vi "ShuffleSplit.vi"(6 "Groups":string[][](array[string]), 8 "error in (no error)":errorcluster caption="entrée d'erreur (pas d'erreur)", 9 "y":string[][](array[string]), 10 "X":string[][](array[string]), 11 "ShuffleSplit":T2={"n_splits"=10, "test_size"="None", "train_size"="None", "random_state"=-1} {"random_state" min=-1}) -> (0 "error out":errorcluster caption="sortie d'erreur", 3 "Split":T1(array[cluster]))   [LabVIEW 2020]
doc: "Random permutation cross-validator\n\nYields indices to split data into training and test sets.\n\nNote: contrary to other cross-validation strategies, random splits do not guarantee that all folds will be different, although this is still very likely for sizeable datasets.\n\n\nParameters :\n\n- n_splits : int, default=10\nNumber of re-shuffling & splitting iterations.\n\n- test_size : float or int, default=None\nIf float, should be between 0.0 and 1.0 and represent the proportion of the dataset to include in the test split. If int, represents the absolute number of test samples. If None, the value is set to the complement of the train size. If train_size is also None, it will be set to 0.1.\n\n- train_size : float or int, default=None\nIf float, should be between 0.0 and 1.0 and represent the proportion of the dataset to include in the train split. If int, represents the absolute number of train samples. If None, the value is automatically set to the complement of the test size.\n\n- random_state : int or RandomState instance, default=None=-1\nControls the randomness of the training and testing indices produced. Pass an int for reproducible output across multiple function calls. \n\n\n\nMethods : Split \n\n\nGenerate indices to split data into training and test set.\n\nParameters : \n\n- X : array-like of shape (n_samples, n_features)\nTraining data, where n_samples is the number of samples and n_features is the number of features.\n\n- y : array-like of shape (n_samples,)\nThe target variable for supervised learning problems.\n\n- groups : array-like of shape (n_samples,), default=None\nGroup labels for the samples used while splitting the dataset into train/test set.\n\nYields : \n\n- train : ndarray\nThe training set indices for that split.\n\n- test : ndarray\nThe testing set indices for that split."
uses:
  ShuffleSplit.lvclass
panel:
  out "ShuffleSplit.lvclass":refnum<class "ShuffleSplit.lvclass">
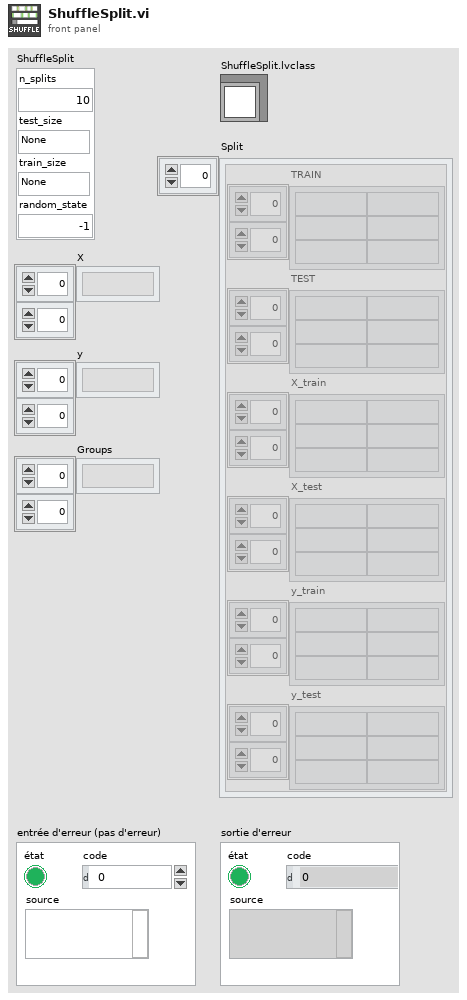
[diagram p1: front panel]
types:
  T1 = cluster{"TRAIN":string[][], "TEST":string[][], "X_train":string[][], "X_test":string[][], "y_train":string[][], "y_test":string[][]}[]
  T2 = cluster{"n_splits":i32, "test_size":string, "train_size":string, "random_state":i32}
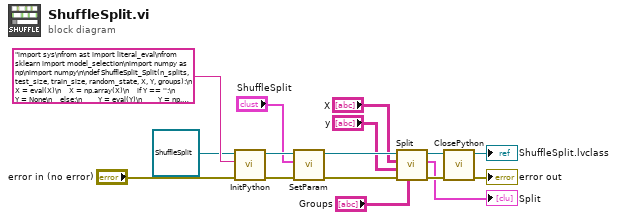
[diagram p0: block diagram]
diagram:
  n1 = call-dynamic "InitPython.vi"("error in (no error)"="error in (no error)", "Python Instruction"="import sys\nfrom ast import literal_eval\nfrom sklearn import model_selection\nimport numpy as np\nimport numpy\n\ndef ShuffleSplit_Split(n_splits, test_size, train_size, random_state, X, Y, groups):\n    X = eval(X)\n    X = np.array(X)\n    if Y == '':\n        Y = None\n    else:\n        Y = eval(Y)\n        Y = np.array(Y)\n    if groups == '':\n        groups = None\n    else:\n        groups = eval(groups)\n        groups = np.array(groups)\n    if test_size == 'None':\n        test_size = None\n    else:\n         test_size = eval(test_size)\n    if train_size == 'None':\n        train_size = None\n    else:\n         train_size = eval(train_size)\n    if random_state == -1:\n        random_state = None\n    list_return = []\n    try:\n        for train_index, test_index in model_selection.ShuffleSplit(n_splits, test_size, train_size, random_state).split(X, Y, groups):\n            list_return = list_return +[\"TRAIN:\", train_index.tolist(), \"TEST:\", test_index.tolist()]\n            X_train, X_test = X[train_index].tolist(), X[test_index].tolist()\n            y_train, y_test = Y[train_index].tolist(), Y[test_index].tolist()\n            list_return = list_return +[\"X_train:\", X_train, \"X_test:\", X_test, \"y_train:\", y_train, \"y_test:\", y_test]\n        return str(list_return)\n    except:\n        erreur = sys.exc_info()\n        typerr = u\"%s\" % (erreur[0])\n        typerr = typerr[typerr.find(\"'\")+1:typerr.rfind(\"'\")]\n        msgerr = u\"%s\" % (erreur[1])\n        message = str('/!\\\\ {0} : {1}'. format(typerr,msgerr))\n        return message", "Scikit-learn en entrée"=refnum<class "ShuffleSplit.lvclass"> refnum ("ShuffleSplit.lvclass")) -> ("error out"=w13:errorcluster, "Scikit-learn en sortie"=w12:refnum<class "ShuffleSplit.lvclass">)  [unwired: 7 in]
  n2 = call-dynamic "SetParam.vi"("error in (no error)"=w13, "ShuffleSplit"="ShuffleSplit", "ShuffleSplit.lvclass"=w12) -> ("error out"=w10:errorcluster, "ShuffleSplit.lvclass"=w9:refnum<class "ShuffleSplit.lvclass">)  [unwired: 7 in]
  n3 = call-dynamic "Split.vi"("Groups"="Groups", "error in (no error)"=w10, "y"="y", "X"="X", "ShuffleSplit.lvclass"=w9) -> ("error out"=w8:errorcluster, "Split"=→"Split":T1, "ShuffleSplit.lvclass"=w7:refnum<class "ShuffleSplit.lvclass">)  [unwired: 4 in]
  n4 = call-dynamic "ClosePython.vi"("error in (no error)"=w8, "Scikit-learn en entrée"=w7) -> ("error out"=→"error out":errorcluster, "Scikit-learn en sortie"=→"ShuffleSplit.lvclass":refnum<class "ShuffleSplit.lvclass">)  [unwired: 8 in]
